vi "UTest_BaselineCorrection.vi"() -> ()   [LabVIEW 2020]
uses:
  SwimDetectParams.ctl
  2a486a1b-0394-4c9c-bf2e-9b099a2067a0.vi
  <vilib>/Analysis/baseanly.llb/Mean (DBL).vi
  <extravilib>/ChannelInstances/Lossy Stream-c(dbl,dbl)/Read With Abort.vi
  <extravilib>/ChannelInstances/Lossy Stream-c(dbl,dbl)/Write With Abort.vi
  <extravilib>/ChannelInstances/Lossy Stream-c(dbl,dbl)/EndpointRead.vi
  <extravilib>/ChannelInstances/Lossy Stream-c(dbl,dbl)/Endpoint.vi
  <extravilib>/ChannelInstances/Lossy Stream-c(dbl,dbl)/Instantiate.vi
  <extravilib>/ChannelInstances/Lossy Stream-c(dbl,dbl)/)Channel.vi
  <resource>/ChannelSupport/_ChannelSupport/WaitIfNeeded.vi
  <vilib>/Utility/file.llb/Read Delimited Spreadsheet (DBL).vi
  <extravilib>/ChannelInstances/Lossy Stream-c(dbl,dbl).lvlib
  <vilib>/Analysis/NI_AALBase.lvlib
panel:
  in  "Control Panel":enum32{"Timing"}(tab)
  in  "No. Samples":i32=300
  in  "Reset Buffers":bool
  in  "Sampling Freq: fs":dbl=100.0 format="%#_13g"
  in  "FY":T1={"U Thresh"=2.5000000000000004, "L Thresh"=-2.5000000000000004, "Driv1 Thresh"=1.0, "Freq Cutoff"=35.0, "STD Scaler"=1.7000000000000004, "Baseline Freq"=0.8999999999999997, "Baseline Scaler"=1.0} {"Freq Cutoff" format="%#_13g"; "Driv1 Thresh" format="%#_13g"}
  in  "TF Data File Path":path
  in  "stop":bool
  out "FY Filtered VR_Update":cluster{dbl, "Filtered Signal":dbl}(graph)
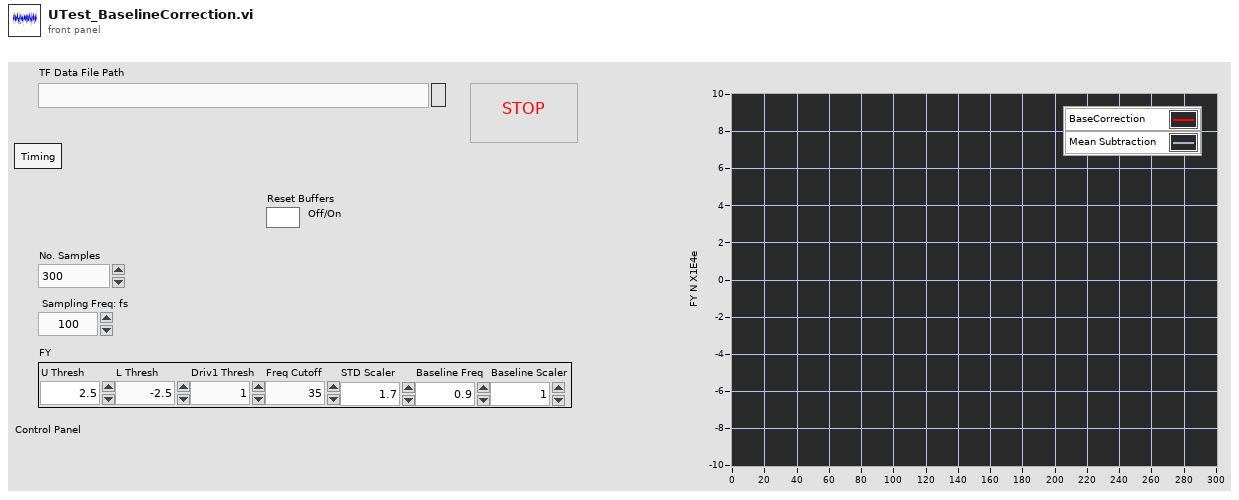
[diagram p1: front panel]
types:
  T1 = typedef "SwimDetectParams.ctl" = cluster{"U Thresh":dbl, "L Thresh":dbl, "Driv1 Thresh":dbl, "Freq Cutoff":dbl, "STD Scaler":dbl, "Baseline Freq":dbl, "Baseline Scaler":dbl}
  T2 = typedef "Lossy Stream-c(dbl,dbl).lvlib/)Channel.ctl" = refnum<queue>
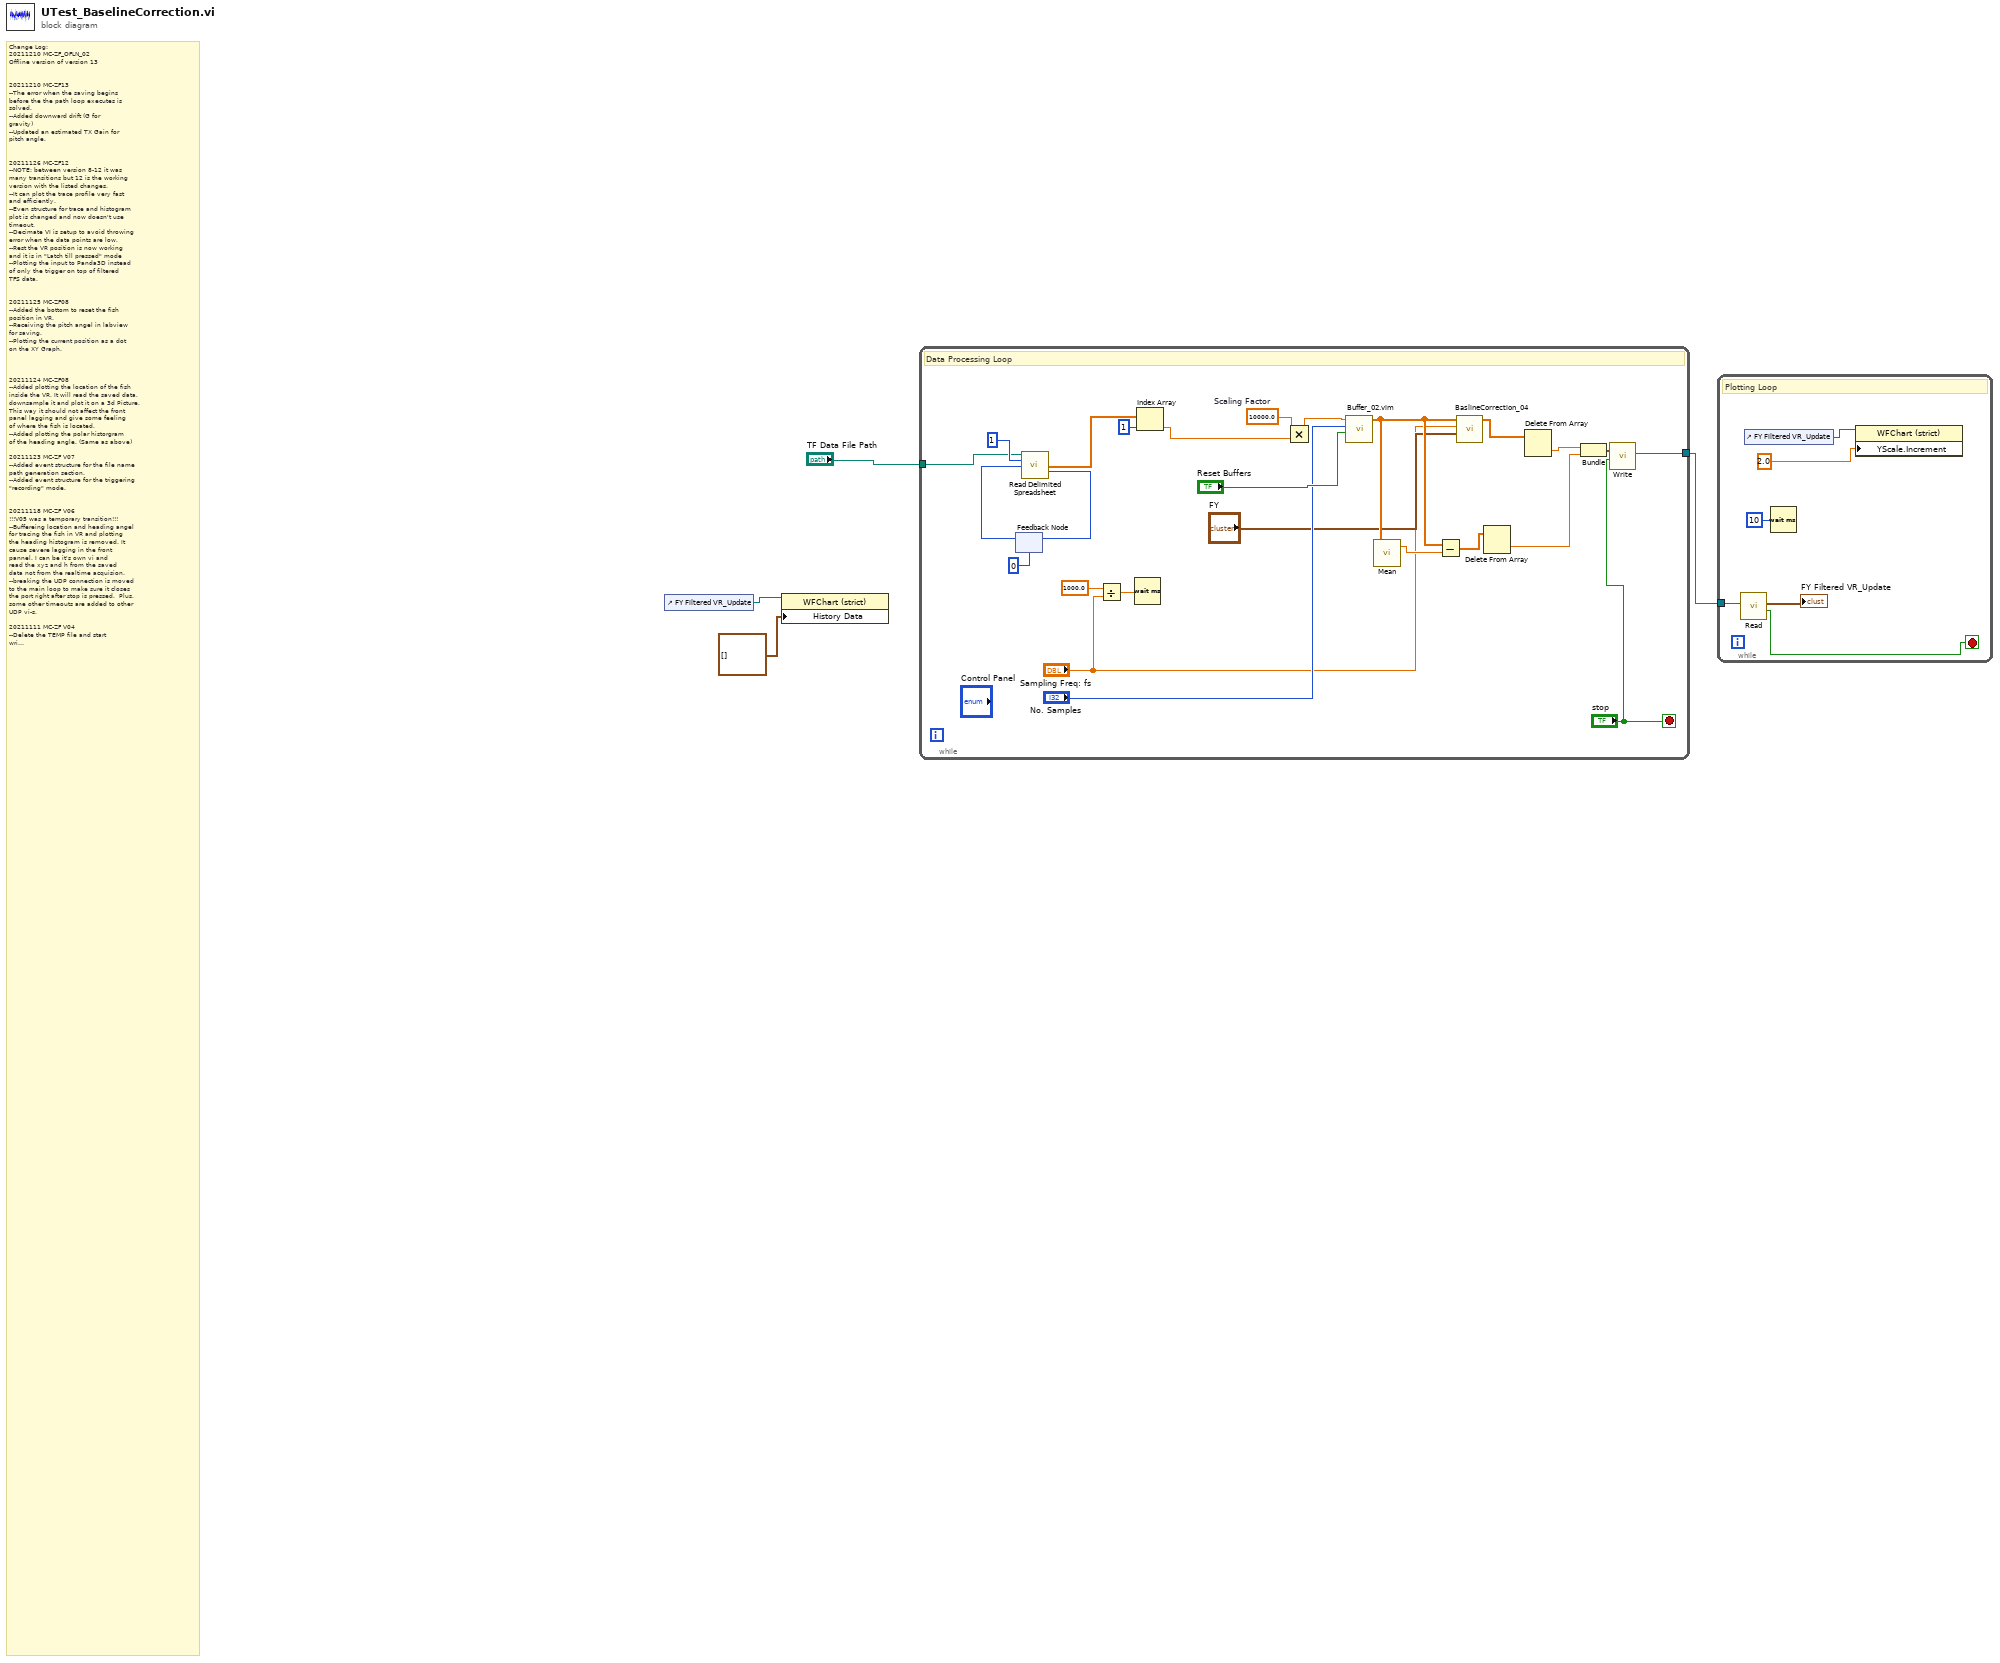
[diagram p0: block diagram]
diagram:
  # "Change Log:\n20211210 MC-ZF_OFLN_02\nOffline version of version 13\n\n\n20211210 MC-ZF13\n--The error when the saving begins\nbefore the the path loop executes is\nsolved. \n--Added downward drift (G for \ngravity)\n--Updated an estimated TX Gain for \npitch angle. \n\n\n20211126 MC-ZF12\n--NOTE: between version 8-12 it was \nmany transitions but 12 is the working \nversion with the listed changes. \n--It can plot the trace profile very fast \nand efficiently.\n--Even structure for trace and histogram \nplot is changed and now doesn't use \ntimeout.\n--Decimate VI is setup to avoid throwing\nerror when the data points are low.\n--Rest the VR position is now working \nand it is in \"Latch till pressed\" mode\n--Plotting the input to Panda3D instead \nof only the trigger on top of filtered \nTFS data. \n\n\n20211125 MC-ZF08\n--Added the bottom to reset the fish \nposition in VR.\n--Receiving the pitch angel in labview \nfor saving.\n--Plotting the current position as a dot\non the XY Graph.\n\n\n\n20211124 MC-ZF08\n--Added plotting the location of the fish\ninside the VR. It will read the saved data, \ndownsample it and plot it on a 3d Picture.\nThis way it should not affect the front \npanel lagging and give some feeling \nof where the fish is located.\n--Added plotting the polar historgram \nof the heading angle. (Same as above)\n\n20211123 MC-ZF V07\n--Added event structure for the file name \npath generation section. \n--Added event structure for the triggering\n\"recording\" mode. \n\n\n20211118 MC-ZF V06\n!!!V05 was a temporary transition!!!\n--Buffereing location and heading angel\nfor tracing the fish in VR and plotting\nthe heading histogram is removed. It \ncause severe lagging in the front\npannel. I can be it's own vi and \nread the xyz and h from the saved \ndata not from the realtime acquision.\n--breaking the UDP connection is moved\nto the main loop to make sure it closes \nthe port right after stop is pressed.  Plus, \nsome other timeouts are added to other \nUDP vi-s. \n\n20211111 MC-ZF V04\n--Delete the TEMP file and start \nwriting to a new TEMP file.\n\n20211104 MC-ZF V03\n--Polishing the UI\n--Changing all the fields to NXG style\n--Removing unnecessary Plots \n--Changing plot style with the trigger \non top of the dara TFS signal\n--VR XYZ in the same channel wire\n\n20211104 MC-ZF V02\n--Save average of all forces and \ntorques \n\n202101102: MC-ZF V01\nFirst online version\nThis VI can \n--trigger Start Acq in ScanImage,\n--count the count the current frame\n--Logs 3 files\n----Averaged LC for FY TX, TZ\n----VR Coordinates with Heading\n----All the parameters on the front \npannel required to reproduce the data \noffline.\n\n\n20210923: V01\nFirst offline version \nthat can read from the TFS data fil and\nmove the camera in Panda3D.\n\nThe data sent to python (Panda3d) \nthrough UDP/IP protocol that will be \ntimed out on either sides if the buffer \nis empty. To avoid getting NAN the \nlast value for each parameter is kept \nis a feedback node to be used.  \n\nTo achive high framerate the \nplotting is rasterized in a different \nloop. The data is passed to the \nplotting loop with a lossy channel \nwire. This type of wire drops data \nif data stream cannot catch up. \n\n\"Last element?\" on the TFS data plot \nis used to stop the plotting loop."
  n1 = control-ref of="FY Filtered VR_Update"() -> (w2:refnum<vi>)
  n2 = property class="WFChart (strict)"(reference=w2, "History Data"=cluster{dbl, "Filtered Signal":dbl}[] []) -> ()  [unwired: 1 in, 2 out]
  n3 = while {
    tunnel: "TF Data File Path" -> [w19]
    tunnel: [w18] -> w3
    stop <- "stop" stop-if-true
    w27 = 10000.0  # Scaling Factor
    # "Data Processing Loop"
    n4 = feedback #1(0 ("mark after read (chars.)")) -> (w23:i32)
    n5 = call-poly <vilib>:"Read Delimited Spreadsheet.vi"("file path (dialog if empty)"=w19, "number of rows (all:-1)"=1, "start of read offset (chars.:0)"=w23) -> ("first row"=w25:dbl[], "mark after read (chars.)"=w24:i32)  [unwired: 7 in, 4 out]
    n6 = feedback-in #1(w24) -> ()
    n7 = Divide(x=1000.0, y="Sampling Freq: fs") -> (x/y=w29:dbl)
    n8 = Wait (ms)(milliseconds to wait=w29) -> ()  [unwired: 1 out]
    n9 = Index Array(array=w25, index=1) -> (element=w20:dbl)
    n10 = Multiply(x=w27, y=w20) -> (x*y=w13:dbl)
    n11 = call "Buffer_02.vim"("Reset"="Reset Buffers", "Max Size"="No. Samples", "New Element"=w13) -> ("Array"=w10:dbl[])  [unwired: 8 in]
    n12 = call-poly <vilib>:"Mean.vi"("X"=w10) -> ("mean"=w9:dbl)  [unwired: 1 out]
    n13 = Subtract(x=w10, y=w9) -> (x-y=w8:dbl[])
    n14 = call "BaslineCorrection_04.vi"("Swim Detect Params"="FY", "Sampling Freq"="Sampling Freq: fs", "Data In"=w10) -> ("Filtered X"=w14:dbl[])  [unwired: 8 in]
    n15 = Delete From Array(array=w8) -> (deleted portion=w7:dbl)  [unwired: 2 in, 1 out]
    n16 = Delete From Array(array=w14) -> (deleted portion=w16:dbl)  [unwired: 2 in, 1 out]
    n17 = Bundle("Numeric"=w16, w7) -> (w11:cluster{"Numeric":dbl, dbl})  [unwired: 1 in]
    n18 = call <extravilib>:"Write.vi"("last element? (F)"="stop", "element"=w11) -> ("channel"=w18:T2)  [unwired: 7 in, 2 out]
  }
  n19 = while {
    tunnel: w3 -> [w34]
    stop <- w33 stop-if-true
    # "Plotting Loop"
    n20 = call <extravilib>:"Read.vi"("channel"=w34) -> ("last element?"=w33:bool, "element"=→"FY Filtered VR_Update":cluster{"Numeric":dbl, "Numeric":dbl})  [unwired: 5 in, 4 out]
    n21 = control-ref of="FY Filtered VR_Update"() -> (w32:refnum<vi>)
    n22 = Wait (ms)(milliseconds to wait=u32 10) -> ()  [unwired: 1 out]
    n23 = property class="WFChart (strict)"(reference=w32, "YScale.Increment"=2.0) -> ()  [unwired: 1 in, 2 out]
  }
